vi "Write_endpointURL.vi"(8 "error in":errorcluster, 10 "Endpoint_URL":string, 11 "URL IN":T1) -> (0 "error out":errorcluster, 3 "URL OUT":T1)   [LabVIEW 2016]
uses:
  URL_Data.ctl
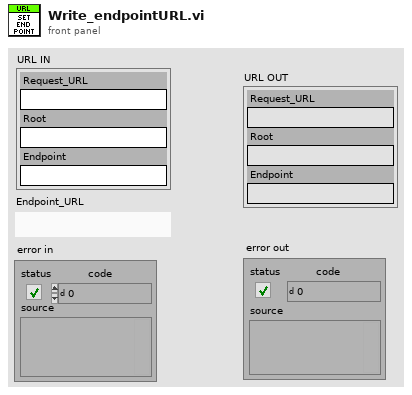
[diagram p1: front panel]
types:
  T1 = typedef "URL_Data.ctl" = cluster{"Root":string, "Endpoint":string, "Request_URL":string}
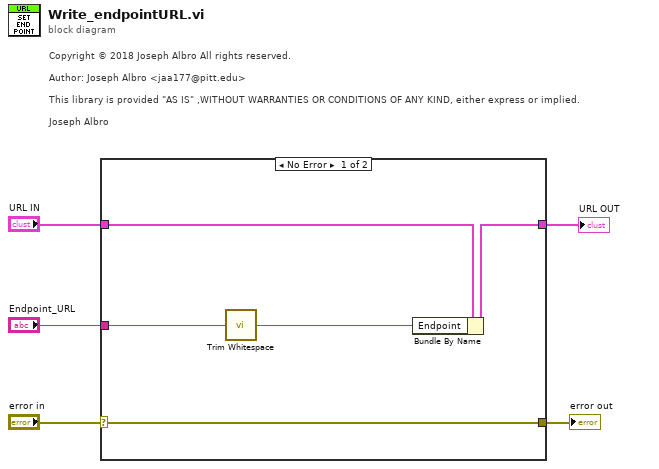
[diagram p0: block diagram]
diagram:
  # "Copyright © 2018 Joseph Albro All rights reserved.\n\nAuthor: Joseph Albro <jaa177@pitt.edu>\n\nThis library is provided \"AS IS\" ,WITHOUT WARRANTIES OR CONDITIONS OF ANY KIND, either express or implied.\n\nJoseph Albro"
  n1 = case shown="No Error" "error in" {
    selector: "error in" -> [w10 w11]
    tunnel: [w10 w11] -> w4
    tunnel: "URL IN" -> [w9 w12]
    tunnel: [w8 w12] -> w2
    tunnel: "Endpoint_URL" -> [w7 _]
    frame No Error {
      n2 = call <vilib>:"Trim Whitespace.vi"("string"=w7) -> ("trimmed string"=w6:string)  [unwired: 1 in]
      n3 = Bundle By Name(cluster=w9, "Endpoint"=w6) -> (w8:T1)
    }
    frame Error {
    }
  }
  "error out" <- w4
  "URL OUT" <- w2
